vi "Faraday status converter.vi"(11 "FC Position":cluster{"IN sensor":bool, "OUT sensor":bool}) -> (3 "FC Status":T1)   [LabVIEW 2016]
doc: "Converts position sensor data to a state:\nFC in (IN sensor = TRUE; OUT sensor = FALSE)\nFC out (IN sensor = FALSE; OUT sensor = TRUE)\nFC status unclear (IN sensor = OUT sensor)"
uses:
  Controls/Faraday cup states.ctl
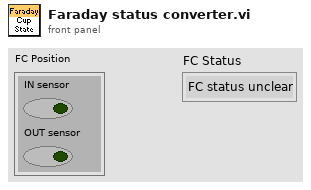
[diagram p1: front panel]
types:
  T1 = typedef "Faraday cup states.ctl" = enum16{"FC status unclear", "FC in", "FC out"}
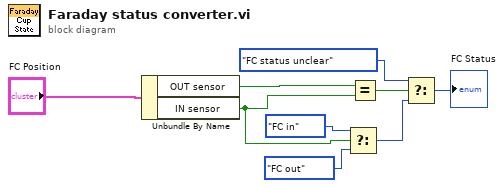
[diagram p0: block diagram]
diagram:
  n1 = Unbundle By Name("FC Position") -> ("OUT sensor"=w2:bool, "IN sensor"=w6:bool)
  n2 = Select(t=Faraday_cup_states."FC in" ("Enum"), s=w6, f=Faraday_cup_states."FC out" ("Enum")) -> (s? t:f=w8:T1)
  n3 = Equal?(x=w2, y=w6) -> (x = y?=w3:bool)
  n4 = Select(t=Faraday_cup_states."FC status unclear" ("Enum"), s=w3, f=w8) -> (s? t:f=→"FC Status":T1)
